vi "CSM - List Sources in Broadcast Registry.vi"(8 "error in (no error)":errorcluster) -> (0 "error out":errorcluster, 3 "Broadcast Names":string[](array[string]))   [LabVIEW 2017, in "Communicable State Machine.lvlib"]
doc: "Lists the broadcast names of all current broadcast registration relationships.\n\n> [!NOTE] \n> <b>CSM Broadcast</b>\n>\n> Broadcasts in CSM are divided into three types: Status Broadcast, Interrupt Broadcast, and State Broadcast. The module pushes the Status Broadcast to all modules registered to that Status Broadcast. Status Broadcast and Interrupt Broadcast are explicitly called broadcasts, while State Broadcast is an implicit broadcast. When a subscription relationship exists, the State Broadcast is automatically triggered when the CSM completes a certain state.\n>\n> - <b>Status Broadcast:</b> Normal priority broadcast. Similar to asynchronous messages, it is passed via the low-priority queue. It is processed sequentially when other unprocessed asynchronous messages or Status Broadcasts exist in the module.\n> - <b>Interrupt Broadcast:</b> High priority broadcast. Similar to synchronous messages, it is passed via the high-priority queue. It is processed first when other low-priority asynchronous messages or Status Broadcasts exist in the module. However, if other unprocessed synchronous messages or Interrupt Broadcasts exist, it is processed sequentially.\n> - <b>State Broadcast:</b> State Broadcast is an implicit broadcast. When a subscription relationship exists, the State Broadcast is automatically triggered when the CSM completes a certain state. The argument for the State Broadcast is the Response of the CSM state.\n\n> [!NOTE] \n> <b>CSM Registration</b>\n>\n> Registration associates a broadcast with a bound interface (API). When the broadcast is triggered, the bound interface (API) is called. Registrations can also be cancelled. In CSM, there are two types of broadcasts:\n>\n> 1. <b>Broadcast:</b> Broadcast explicitly called by the module sending the broadcast message. Arguments need to be explicitly provided.\n> 2. <b>State:</b> Any state of a CSM module can also be registered to. The argument received by the triggered API is the Response of the CSM state.\n>\n> // Register `[Broadcast Message Name]@[SourceModule] >> [Bound API]@[TargetModule] -><register> // [Comments]`// Unregister `[Broadcast Message Name]@[SourceModule] >> [Bound API]@[TargetModule] -><unregister> // [Comments]`\n\n> - <b>Broadcast Message Name:</b> Defined by the source module. Refer to \"CSM Broadcast Format Parsing\" for details.\n> - <b>Source Module:</b> The broadcasting module. If subscribing to broadcasts from any module, the source module can be represented by `*`.\n> - <b>Bound API:</b> Defined by the target module. It is the external interface of the target module.\n> - <b>Target Module:</b> The module where the bound API resides. When indicating registration to the current module within a CSM module, it can be ignored. The preceding `@` separator is also omitted.\n> - `<register>` / `<unregister>`: Definition of the Register/Unregister operation type.\n> - <b>Comments:</b> Comment information, which will not be parsed.\n\n-- <b>Indicators</b> --\n- <b>Broadcast Names</b>: Broadcast names of all current broadcast registration relationships."
uses:
  Communicable State Machine.lvlib
  _Support/FGV-BroadcastRegistry/Operation-BroadcastRegistry.ctl
  _Support/ChangeFlag/ChangeFlag-Read.vi
  _Support/ChangeFlag/ChangeFlagDB.vi
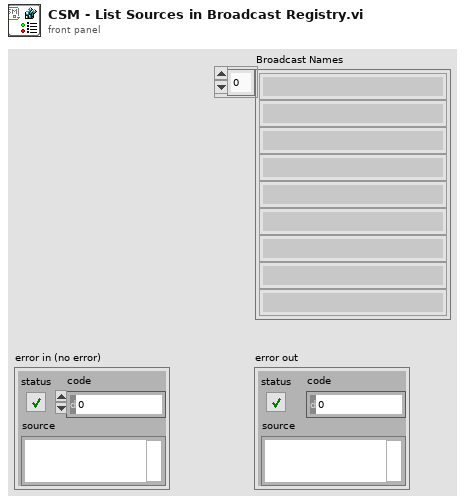
[diagram p1: front panel]
types:
  T1 = typedef "Communicable State Machine.lvlib/Operation-BroadcastRegistry.ctl" = enum16{"Delete Source Module", "Delete Target Module", "Remove Module", "Register", "Unregister", "Check", "List Status", "List Entries", "List Status Of Source", "Drop", "Register As Status", "Register As Interrupt"}
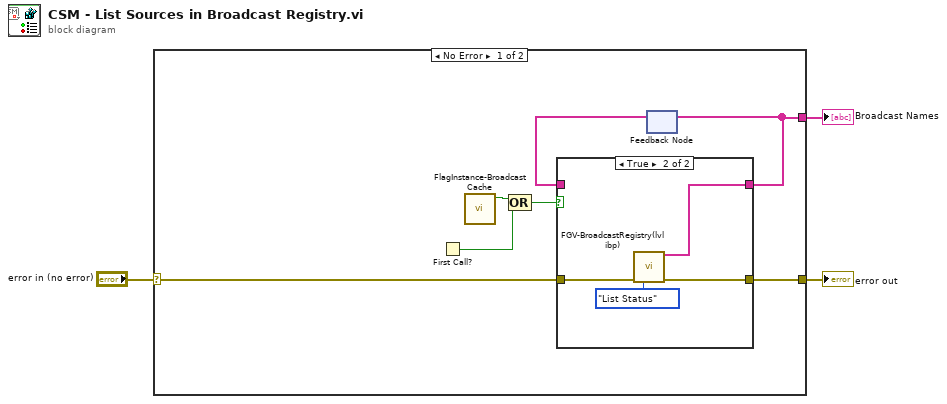
[diagram p0: block diagram]
diagram:
  n1 = case shown="No Error" "error in (no error)" {
    selector: "error in (no error)" -> [w10 w17]
    tunnel: [w7 _] -> w2
    tunnel: [w5 w17] -> w1
    frame No Error {
      n2 = First Call?() -> (First Call?: T/F=w9:bool)
      n3 = call "FlagInstance-Broadcast Cache.vi"() -> ("Changed"=w4:bool)  [unwired: 10 in, 1 out]
      n4 = Compound Arithmetic op=OR(w4, w9) -> (w8:bool)
      n5 = feedback #1() -> (w6:string[])  [unwired: 1 in]
      n6 = case shown="True" w8 {
        tunnel: [w12 w16] -> w5
        tunnel: w10 -> [w12 w15]
        tunnel: [w11 w13] -> w7
        tunnel: w6 -> [w11 _]
        frame False {
        }
        frame True {
          n7 = call "FGV-BroadcastRegistry(lvlibp).vi"("Error In"=w15, "Operation"=Operation-BroadcastRegistry."List Status") -> ("Response Message"=w13:string[], "error out"=w16:errorcluster)  [unwired: 11 in, 1 out]
        }
      }
      n8 = feedback-in #1(w7) -> ()
    }
    frame Error {
    }
  }
  "error out" <- w1
  "Broadcast Names" <- w2
